vi "Track the Maximum Temperature.vi"() -> ()   [LabVIEW 2020]
uses:
  <vilib>/DAQmx/read.llb/DAQmx Read (Analog DBL 1Chan 1Samp).vi
  <vilib>/DAQmx/create/channels.llb/DAQmx Create Channel (AI-Temperature-Thermocouple).vi
  <vilib>/DAQmx/configure/timing.llb/DAQmx Timing (Sample Clock).vi
  <vilib>/DAQmx/miscellaneous.llb/DAQmx Fill In Error Info.vi
panel:
  out "Max Temperature Acquired (deg C)":dbl
  in  "Stop":bool
  out "Temperature Chart":dbl(graph)
  in  "Thermocouple Channel":tag="PCI-6221/ai0"
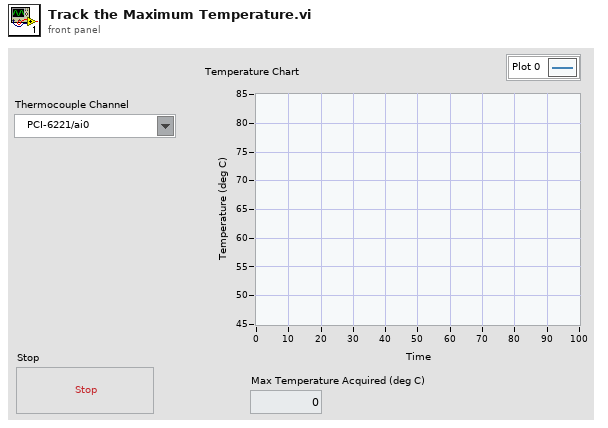
[diagram p1: front panel]
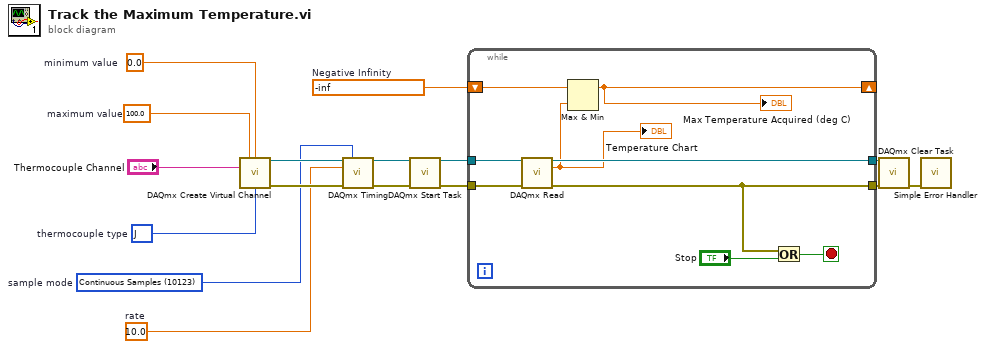
[diagram p0: block diagram]
diagram:
  w1 = -inf  # Negative Infinity
  w10 = 10072 items=["J"=10072, "K"=10073, "N"=10077, "R"=10082, "S"=10085, "T"=10086, "B"=10047, "E"=10055]  # thermocouple type
  w11 = 0.0  # minimum value
  w12 = 100.0  # maximum value
  w13 = 10.0  # rate
  w14 = 10123 items=["Finite Samples"=10178, "Continuous Samples"=10123, "Hardware Timed Single Point"=12522]  # sample mode
  n1 = call-poly <vilib>:"DAQmx Create Virtual Channel.vi"("maximum value"=w12, "minimum value"=w11, "physical channels"="Thermocouple Channel", "thermocouple type"=w10) -> ("task out"=w16:refnum<k21>, "error out"=w15:errorcluster)  [unwired: 10 in]
  n2 = call-poly <vilib>:"DAQmx Timing.vi"("task/channels in"=w16, "sample mode"=w14, "rate"=w13, "error in"=w15) -> ("task out"=w8:refnum<k21>, "error out"=w7:errorcluster)  [unwired: 10 in]
  n3 = call <vilib>:"DAQmx Start Task.vi"("task/channels in"=w8, "error in"=w7) -> ("task out"=w6:refnum<k21>, "error out"=w5:errorcluster)  [unwired: 12 in]
  n4 = while {
    tunnel: w6 -> [w25]
    tunnel: [w23] -> w4
    tunnel: w5 -> [w24]
    tunnel: [w22] -> w3
    shift-right: [w17] -> _
    shift-left: w1 -> [w19]
    stop <- w21 stop-if-true
    n5 = call-poly <vilib>:"DAQmx Read.vi"("task/channels in"=w25, "error in"=w24) -> ("task out"=w23:refnum<k21>, "data"=w18:dbl, "error out"=w22:errorcluster)  [unwired: 11 in]
    "Temperature Chart" <- w18
    n6 = Max & Min(x=w19, y=w18) -> (max(x,y)=w17:dbl)  [unwired: 1 out]
    "Max Temperature Acquired (deg C)" <- w17
    n7 = Or(x=w22, y="Stop") -> (x .or. y?=w21:bool)
  }
  n8 = call <vilib>:"DAQmx Clear Task.vi"("task in"=w4, "error in"=w3) -> ("error out"=w2:errorcluster)  [unwired: 13 in]
  n9 = call <vilib>:"Simple Error Handler.vi"("error in (no error)"=w2) -> ()  [unwired: 4 in, 5 out]
